vi "Read Method.vi"(11 "Switching Time in":refnum<class "Switching Time.lvclass">) -> (2 "Method":T1, 3 "Switching Time out":refnum<class "Switching Time.lvclass">)   [LabVIEW 2020, in "Switching Time.lvclass"]
uses:
  Switching Time.lvclass
  Controls/Method.ctl
  Switching Time.lvclass/Switching Time.ctl
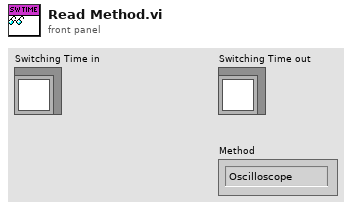
[diagram p1: front panel]
types:
  T1 = typedef "Switching Time.lvclass/Method.ctl" = enum16{"Oscilloscope", "Spectrum Analyzer"}
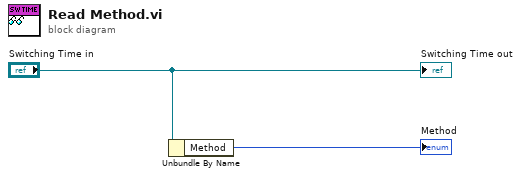
[diagram p0: block diagram]
diagram:
  n1 = Unbundle By Name("Switching Time in") -> ("Method"=→"Method":enum16{"Oscilloscope", "Spectrum Analyzer"})
  "Switching Time out" <- "Switching Time in"
